vi "Open Arm.vi"(8 "error in (no error)":errorcluster) -> (0 "error out 2":errorcluster)   [LabVIEW 2018]
uses:
  TypeDefs/typedef_enum_Refnums.ctl
  <vilib>/Rock Robotics/WPI/ThirdParty/Phoenix-LabVIEW/Motor Controller/Controls/CTRE_Phoenix_MotorControl_FeedbackDevice.ctl
  <vilib>/Rock Robotics/WPI/ThirdParty/Phoenix-LabVIEW/Pigeon IMU/CTRE_PigeonIMU_Open_TalonSRX.vi
panel:
  in  "error in (no error) 2":errorcluster
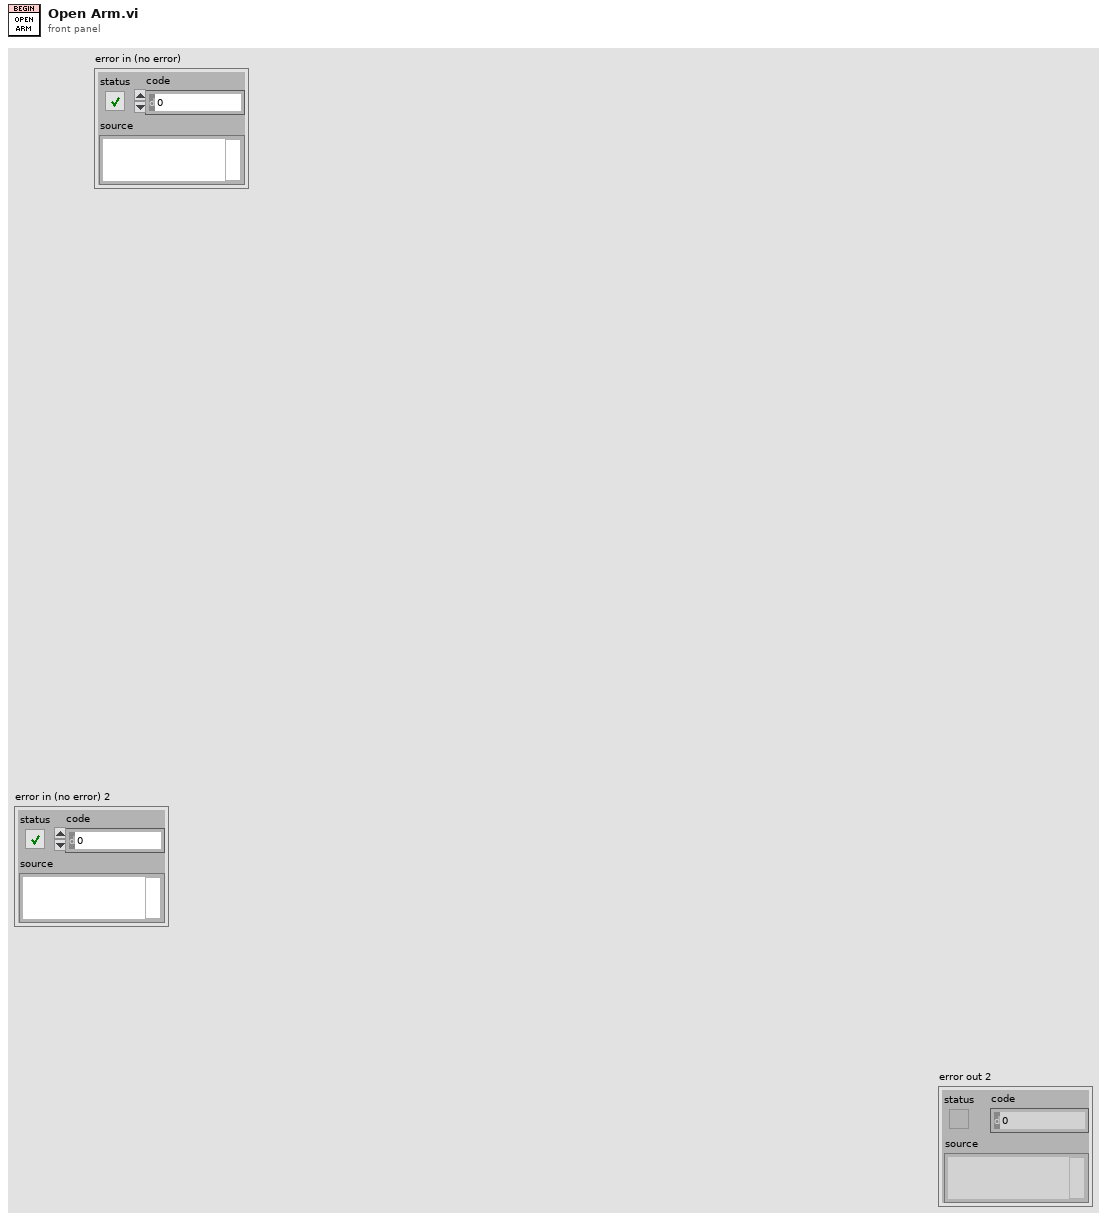
[diagram p1: front panel]
types:
  T1 = typedef "CTRE_Phoenix_MotorControl_FeedbackDevice.ctl" = i8
  T2 = typedef "typedef_enum_Refnums.ctl" = enum16{"Ball_Encoder", "Ball_Motor", "Camera", "Linefollow_3", "Linefollow_2", "Linefollow_1", "Gyro", "Hatch_Solenoid", "Climb_Back_Solenoid", "Arm_Encoder", "Arm_Motor", "Lift_Encoder", "Drive", "Drive_Motor_R", "Drive_Motor_L", "Drive_Encoder_R", "Drive_Encoder_L", "Joy_R", "Joy_L", "Wrist_Motor", "Wrist_Encoder", "Climb Upper Limit", "Climb Lower Limit ", "Climb_Front_Motor"}
  T3 = typedef "typedef_enum_Refnums.ctl" = enum16{"Ball_Encoder", "Ball_Motor", "Camera", "Linefollow_3", "Linefollow_2", "Linefollow_1", "Gyro", "Hatch_Solenoid", "Climb_Back_Solenoid", "Arm_Encoder", "Arm_Motor", "Lift_Encoder", "Arm_Motor_R", "Arm_Motor_L", "Drive", "Drive_Motor_R", "Drive_Motor_L", "Drive_Encoder_R", "Drive_Encoder_L", "Joy_R", "Joy_L", "Wrist_Motor", "Wrist_Encoder", "Climb_Front_Encoder", "Climb_Front_Motor"}
  T4 = typedef "WPI_MotorControlDeviceRef.ctl" = cluster{"DeviceStatus":errorcluster, "Type":T5, "PWM":cluster{"PWM Channel":T6, "DeadBand":T7}, "CAN":cluster{"Device Number":u8, "SetOutput VI Ref":variant, "GetOutput VI Ref":variant, "Enable VI Ref":variant, "Disable VI Ref":variant, "Data":variant}, "Invert":bool, "DIO PWM":cluster{"PWM \"Enable\" Channel":T6, "DIOChannel":T8, "PWM Rate":dbl}}
  T5 = typedef "WPI_MotorControlType.ctl" = enum16{"PWM", "CAN", "DIO PWM"}
  T6 = typedef "FPGA_DIOPWMChannel.ctl" = enum8{"PWM 0", "PWM 1", "PWM 2", "PWM 3", "PWM 4", "PWM 5", "PWM 6", "PWM 7", "PWM 8", "PWM 9", "PWM MXP 0", "PWM MXP 1", "PWM MXP 2", "PWM MXP 3", "PWM MXP 4", "PWM MXP 5", "PWM MXP 6", "PWM MXP 7", "PWM MXP 8", "PWM MXP 9", "Invalid"}
  T7 = typedef "WPI_PWMDeadband.ctl" = cluster{"Name":string, "maxPositivePwm":i32, "minPositivePwm":i32, "centerPwm":i32, "maxNegativePwm":i32, "minNegativePwm":i32, "angularRange":u16}
  T8 = typedef "FPGA_DIOChannel.ctl" = enum8{"DIO 0", "DIO 1", "DIO 2", "DIO 3", "DIO 4", "DIO 5", "DIO 6", "DIO 7", "DIO 8", "DIO 9", "DIO MXP 0", "DIO MXP 1", "DIO MXP 2", "DIO MXP 3", "DIO MXP 4", "DIO MXP 5", "DIO MXP 6", "DIO MXP 7", "DIO MXP 8", "DIO MXP 9", "DIO MXP 10", "DIO MXP 11", "DIO MXP 12", "DIO MXP 13", "DIO MXP 14", "DIO MXP 15", "SPI Port CS1", "SPI Port CS2", "SPI Port CS3", "SPI Port MISO", "SPI Port MOSI", "Invalid"}
  T9 = typedef "CTRE_PigeonIMU_DeviceRef.ctl" = cluster{"DeviceStatus":errorcluster, "Device Number":u8, "Type":T10, "Device ID":u32, "Handle":u64, "UsageFrame":u32, "Library Path":path}
  T10 = typedef "CTRE_PigeonIMU_ConnectionType.ctl" = u32
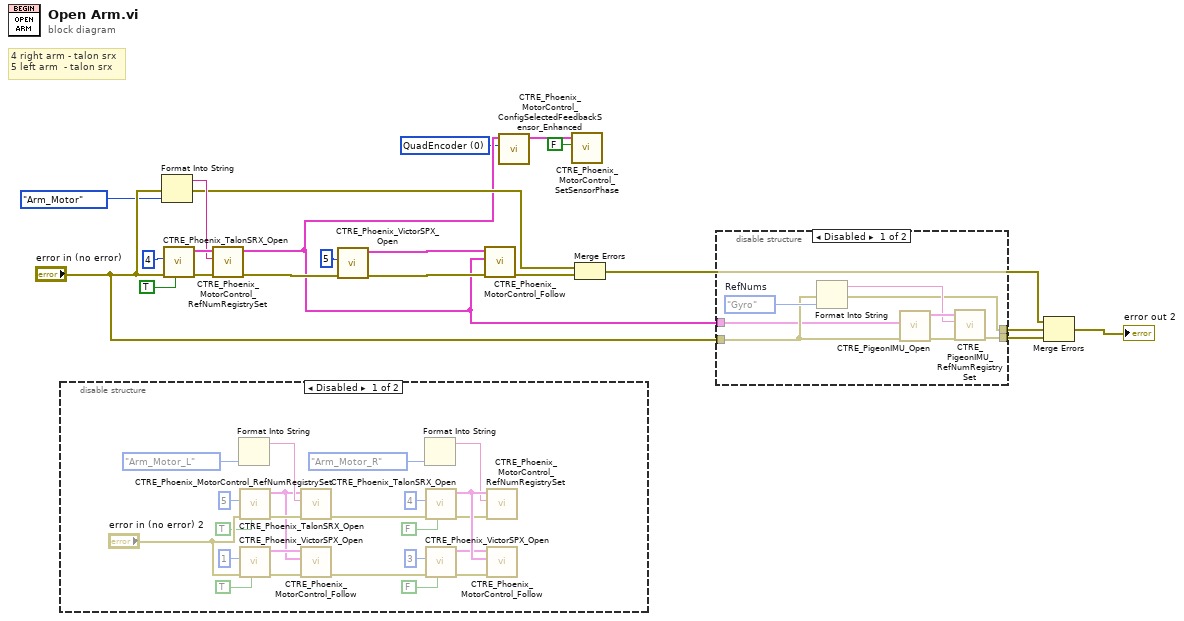
[diagram p0: block diagram]
diagram:
  w2 = T1 0 items=["QuadEncoder"=0, "Analog"=2, "Tachometer"=4, "Pulse Width Encoded Position"=8, "Sensor Sum (S0 + S1)"=9, "Sensor Difference (D0 - D1)"=10, "Remote Source 0"=11, "Remote Source 1"=12, "Software Emulated"=15] ("Feedback Device")
  # "4 right arm - talon srx\n5 left arm  - talon srx"
  n1 = disable-structure shown="Disabled" {
    frame Disabled {
      n2 = Format Into String(typedef_enum_Refnums."Arm_Motor_L" ("RefNums")) -> (resulting string=w43:string)  [unwired: 3 in, 1 out]
      n3 = call <vilib>:"CTRE_Phoenix_TalonSRX_Open.vi"("Invert"=TRUE, "error in"="error in (no error) 2", "Device Number"=u8 5) -> ("error out"=w45:errorcluster, "CAN Talon SRX Ref"=w39:T4)  [unwired: 7 in]
      n4 = call <vilib>:"CTRE_Phoenix_VictorSPX_Open.vi"("Invert"=TRUE, "error in"="error in (no error) 2", "Device Number"=u8 1) -> ("error out"=w41:errorcluster, "CAN Talon SRX Ref"=w40:T4)  [unwired: 7 in]
      n5 = call <vilib>:"CTRE_Phoenix_MotorControl_RefNumRegistrySet.vi"("error in (no error)"=w45, "refnum name"=w43, "PhoenixMotorControlDevRef"=w39) -> ("error out"=w28:errorcluster, "PhoenixMotorControlDevRef"=w22:T4)  [unwired: 7 in]
      n6 = call <vilib>:"CTRE_Phoenix_MotorControl_Follow.vi"("error in (no error)"=w41, "Master Controller to Follow"=w39, "PhoenixMotorControlDevRef"=w40) -> ("error out"=w27:errorcluster)  [unwired: 7 in, 1 out]
      n7 = Format Into String(typedef_enum_Refnums."Arm_Motor_R" ("RefNums")) -> (resulting string=w32:string)  [unwired: 3 in, 1 out]
      n8 = call <vilib>:"CTRE_Phoenix_TalonSRX_Open.vi"("Invert"=FALSE, "error in"=w28, "Device Number"=u8 4) -> ("error out"=w30:errorcluster, "CAN Talon SRX Ref"=w36:T4)  [unwired: 7 in]
      n9 = call <vilib>:"CTRE_Phoenix_VictorSPX_Open.vi"("Invert"=FALSE, "error in"=w27, "Device Number"=u8 3) -> ("error out"=w34:errorcluster, "CAN Talon SRX Ref"=w35:T4)  [unwired: 7 in]
      n10 = call <vilib>:"CTRE_Phoenix_MotorControl_RefNumRegistrySet.vi"("error in (no error)"=w30, "refnum name"=w32, "PhoenixMotorControlDevRef"=w36) -> ()  [unwired: 7 in, 2 out]
      n11 = call <vilib>:"CTRE_Phoenix_MotorControl_Follow.vi"("error in (no error)"=w34, "Master Controller to Follow"=w36, "PhoenixMotorControlDevRef"=w35) -> ()  [unwired: 7 in, 2 out]
    }
    frame Enabled {
    }
  }
  n12 = Format Into String(error in="error in (no error)", typedef_enum_Refnums."Arm_Motor" ("RefNums")) -> (resulting string=w19:string, error out=w13:errorcluster)  [unwired: 2 in]
  n13 = call <vilib>:"CTRE_Phoenix_TalonSRX_Open.vi"("Invert"=TRUE, "error in"="error in (no error)", "Device Number"=u8 4) -> ("error out"=w21:errorcluster, "CAN Talon SRX Ref"=w20:T4)  [unwired: 7 in]
  n14 = call <vilib>:"CTRE_Phoenix_MotorControl_RefNumRegistrySet.vi"("error in (no error)"=w21, "refnum name"=w19, "PhoenixMotorControlDevRef"=w20) -> ("error out"=w14:errorcluster, "PhoenixMotorControlDevRef"=w3:T4)  [unwired: 7 in]
  n15 = call <vilib>:"CTRE_Phoenix_VictorSPX_Open.vi"("error in"=w14, "Device Number"=u8 5) -> ("error out"=w18:errorcluster, "CAN Talon SRX Ref"=w17:T4)  [unwired: 8 in]
  n16 = call <vilib>:"CTRE_Phoenix_MotorControl_Follow.vi"("error in (no error)"=w18, "Master Controller to Follow"=w3, "PhoenixMotorControlDevRef"=w17) -> ("error out"=w12:errorcluster)  [unwired: 7 in, 1 out]
  n17 = call <vilib>:"CTRE_Phoenix_MotorControl_ConfigSelectedFeedbackSensor_Enhanced.vi"("Feedback Device"=w2, "PhoenixMotorControlDevRef"=w3) -> ("PhoenixMotorControlDevRef"=w5:T4)  [unwired: 8 in, 1 out]
  n18 = call <vilib>:"CTRE_Phoenix_MotorControl_SetSensorPhase.vi"("PhaseSensor"=FALSE, "PhoenixMotorControlDevRef"=w5) -> ()  [unwired: 8 in, 2 out]
  n19 = Merge Errors(w13, w12) -> (w7:errorcluster)
  n20 = disable-structure shown="Disabled" {
    disable-tunnel: [w49 _] -> w9
    disable-tunnel: [w48 _] -> w8
    disable-tunnel: "error in (no error)" -> [w47 _]
    disable-tunnel: w3 -> [w46 _]
    frame Disabled {
      w51 = typedef_enum_Refnums."Gyro"  # RefNums
      n21 = Format Into String(error in=w47, w51) -> (resulting string=w50:string, error out=w48:errorcluster)  [unwired: 2 in]
      n22 = call-poly <vilib>:"CTRE_PigeonIMU_Open.vi"("error in"=w47, "CAN Talon SRX Ref"=w46) -> ("error out"=w52:errorcluster, "PigeonIMUDevRef"=w53:T9)  [unwired: 8 in]
      n23 = call <vilib>:"CTRE_PigeonIMU_RefNumRegistrySet.vi"("error in (no error)"=w52, "refnum name"=w50, "PigeonIMUDevRef"=w53) -> ("error out"=w49:errorcluster)  [unwired: 7 in, 1 out]
    }
    frame Enabled {
    }
  }
  n24 = Merge Errors(w7, w8, w9) -> (→"error out 2":errorcluster)
